vi "SLL DE AO Min Max Range Checking.vi"(4 "Analog Output Channels":refnum<k21>[](array[refnum]), 6 "AO Values In":dbl[](array[numeric]), 7 "Option":T2=enum."Check Single AO Channel", 8 "error in (no error)":errorcluster, 9 "AO Channels Name":T1[](array[typedef]), 10 "AO Value":dbl, 11 "AO Channel Name":T1) -> (0 "error out":errorcluster, 2 "AO Values Out":dbl[](array[numeric]), 3 "AO Value Out":dbl)   [LabVIEW 2013]
uses:
  Controls/SLL DE AO Min Max Range Checking Options.ctl
  Controls/SLL DE List of Analog Outputs.ctl
  <resource>/objmgr/daqmx.rc
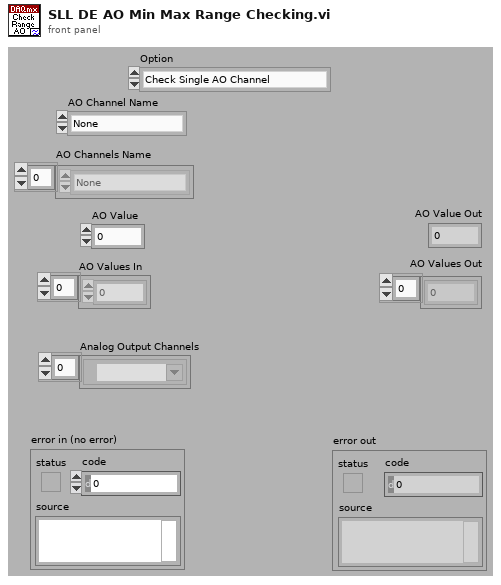
[diagram p1: front panel]
types:
  T1 = typedef "SLL DE List of Analog Outputs.ctl" = enum16{"None"}
  T2 = typedef "SLL DE AO Min Max Range Checking Options.ctl" = enum16{"Initalize Channel Range", "Check Single AO Channel", "Check Multiple AO Channels"}
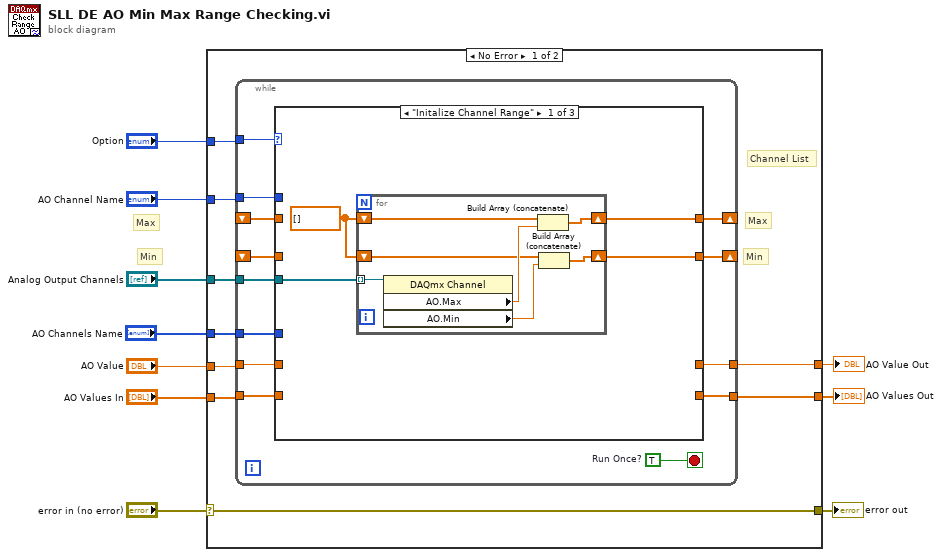
[diagram p0: block diagram]
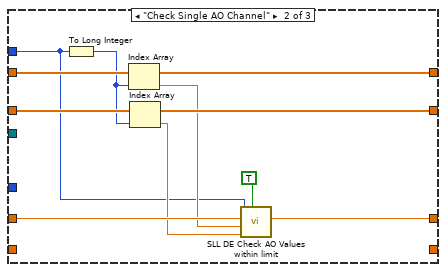
[diagram p2: hidden frame]
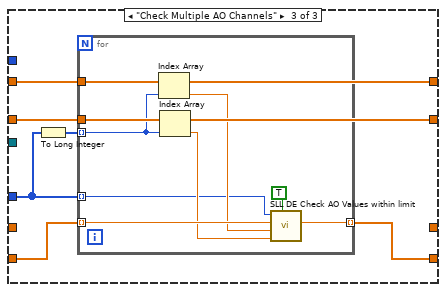
[diagram p3: hidden frame]
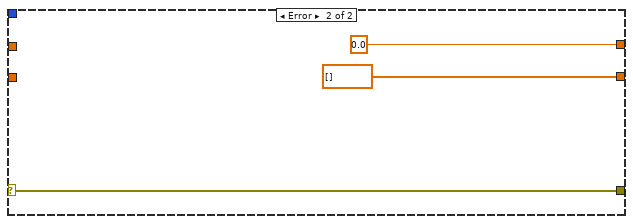
[diagram p4: hidden frame]
diagram:
  # "Max"
  # "Min"
  n1 = case shown="No Error" "error in (no error)" {
    selector: "error in (no error)" -> [w12 w70]
    tunnel: "Analog Output Channels" -> [w19 _]
    tunnel: "Option" -> [w18 _]
    tunnel: "AO Channel Name" -> [w17 _]
    tunnel: "AO Value" -> [w16 _]
    tunnel: [w15 0.0 ("value")] -> w6
    tunnel: "AO Values In" -> [w14 _]
    tunnel: [w13 dbl[] []] -> w4
    tunnel: [w12 w70] -> w2
    tunnel: "AO Channels Name" -> [w11 _]
    frame No Error {
      # "Channel List"
      # "Max"
      # "Min"
      n2 = while {
        tunnel: w19 -> [w32]
        tunnel: w18 -> [w30]
        shift-right: [w29] -> _
        shift-left: _ -> [w27]
        shift-right: [w28] -> _
        shift-left: _ -> [w26]
        tunnel: w17 -> [w25]
        tunnel: w16 -> [w24]
        tunnel: [w23] -> w15
        tunnel: w14 -> [w22]
        tunnel: [w21] -> w13
        tunnel: w11 -> [w20]
        stop <- w31 stop-if-true
        w31 = TRUE  # Run Once?
        n3 = case shown="\"Initalize Channel Range\"" w30 {
          tunnel: w32 -> [w34 _ _]
          tunnel: [w36 w48 w57] -> w29
          tunnel: [w35 w50 w58] -> w28
          tunnel: w27 -> [_ w48 w57]
          tunnel: w26 -> [_ w50 w58]
          tunnel: w25 -> [_ w45 _]
          tunnel: w24 -> [_ w51 _]
          tunnel: [_ w46 _] -> w23
          tunnel: w22 -> [_ _ w56]
          tunnel: [_ _ w55] -> w21
          tunnel: w20 -> [_ _ w53]
          frame "Initalize Channel Range" {
            w33 = dbl[] []
            n4 = for {
              shift-right: [w41] -> w36
              shift-left: w33 -> [w39]
              tunnel: w34 -> [w37] mode=indexing
              shift-right: [w40] -> w35
              shift-left: w33 -> [w38]
              n5 = property class="DAQmx Channel"(reference=w37) -> ("AO.Max"=w43:dbl, "AO.Min"=w42:dbl)  [unwired: 1 in, 2 out]
              n6 = Build Array (concatenate)(w39, w43) -> (w41:dbl[])
              n7 = Build Array (concatenate)(w38, w42) -> (w40:dbl[])
            }
          }
          frame "Check Single AO Channel" {
            n8 = To Long Integer(number=w45) -> (32bit integer=w44:i32)
            n9 = Index Array(array=w48, index=w44) -> (element=w47:dbl)
            n10 = Index Array(array=w50, index=w44) -> (element=w49:dbl)
            n11 = call "SLL DE Check AO Values within limit.vi"("Display Dialog"=TRUE, "AO Min Values"=w49, "AO Max Values"=w47, "AO Value"=w51, "AO Channel Name"=w45) -> ("value"=w46:dbl)  [unwired: 6 in]
          }
          frame "Check Multiple AO Channels" {
            n12 = To Long Integer(number=w53) -> (32bit integer=w54:i32[])
            n13 = for {
              tunnel: w56 -> [w66] mode=indexing
              tunnel: w54 -> [w60] mode=indexing
              tunnel: w58 -> [w65]
              tunnel: w57 -> [w63]
              tunnel: [w61] -> w55 mode=indexing
              tunnel: w53 -> [w59] mode=indexing
              n14 = Index Array(array=w63, index=w60) -> (element=w62:dbl)
              n15 = Index Array(array=w65, index=w60) -> (element=w64:dbl)
              n16 = call "SLL DE Check AO Values within limit.vi"("Display Dialog"=TRUE, "AO Min Values"=w64, "AO Max Values"=w62, "AO Value"=w66, "AO Channel Name"=w59) -> ("value"=w61:dbl)  [unwired: 6 in]
            }
          }
        }
      }
    }
    frame Error {
    }
  }
  "AO Value Out" <- w6
  "AO Values Out" <- w4
  "error out" <- w2
